vi "FTW-Request-WriteResponse.vi"(0 "FTW Incoming Request":refnum<class "FTW-Request.lvclass">, 5 "Response Body":string, 11 "error in":errorcluster) -> (4 "FTW Incoming Request out":refnum<class "FTW-Request.lvclass">, 15 "error out":errorcluster)   [LabVIEW 2014, in "FTW-Request.lvclass"]
uses:
  FTW-Request.lvclass
  FTW-Request.lvclass/FTW-Request.ctl
panel:
  # "Inputs"
  # "Outputs"
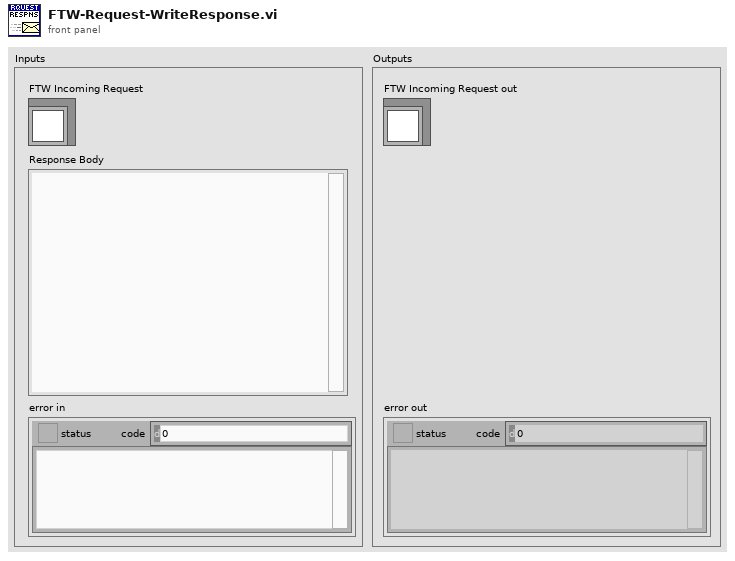
[diagram p1: front panel]
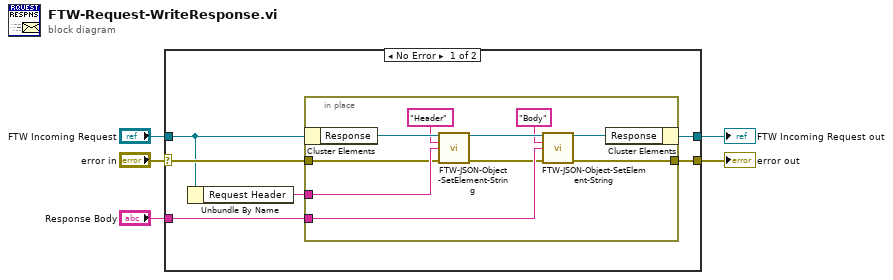
[diagram p0: block diagram]
diagram:
  n1 = case shown="No Error" "error in" {
    selector: "error in" -> [w9 w22]
    tunnel: [w8 w22] -> w4
    tunnel: [w11 w23] -> w3
    tunnel: "FTW Incoming Request" -> [w7 w23]
    tunnel: "Response Body" -> [w10 _]
    frame No Error {
      n2 = Unbundle By Name(w7) -> ("Request Header"=w6:string)
      n3 = in-place {
        in-place-border: w6 -> [w17]
        in-place-border: w10 -> [w16]
        in-place-border: w9 -> [w14]
        in-place-border: [w12] -> w8
        n4 = in-place-cluster #1(w7) -> ("Response"=w21:refnum<data-value>)
        n5 = call "FTW-JSON-Object-SetElement-String.vi"("JSON Object"=w21, "Key"="Header", "Value"=w17, "error in"=w14) -> ("JSON Object out"=w20:refnum<data-value>, "error out"=w13:errorcluster)  [unwired: 10 in]
        n6 = call "FTW-JSON-Object-SetElement-String.vi"("JSON Object"=w20, "Key"="Body", "Value"=w16, "error in"=w13) -> ("JSON Object out"=w19:refnum<data-value>, "error out"=w12:errorcluster)  [unwired: 10 in]
        n7 = in-place-cluster #1("Response"=w19) -> (w11:refnum<class "FTW-Request.lvclass">)
      }
    }
    frame Error {
    }
  }
  "error out" <- w4
  "FTW Incoming Request out" <- w3
